vi "gyro calibration.vi"() -> ()   [LabVIEW 2012]
panel:
  in  "退出程序":bool caption="停止电机 2"
  out "角速度(deg/s)":dbl
  out "相对偏角(deg)":dbl(graph)
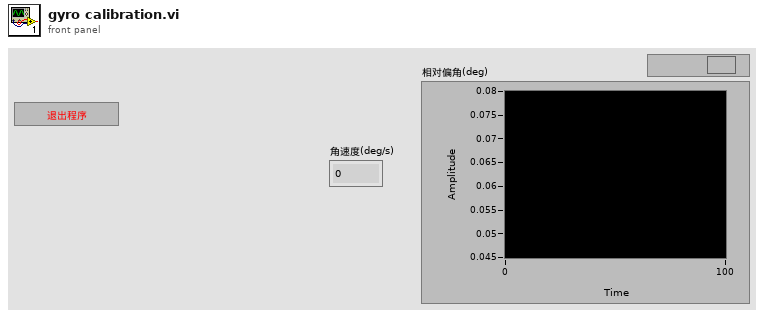
[diagram p1: front panel]
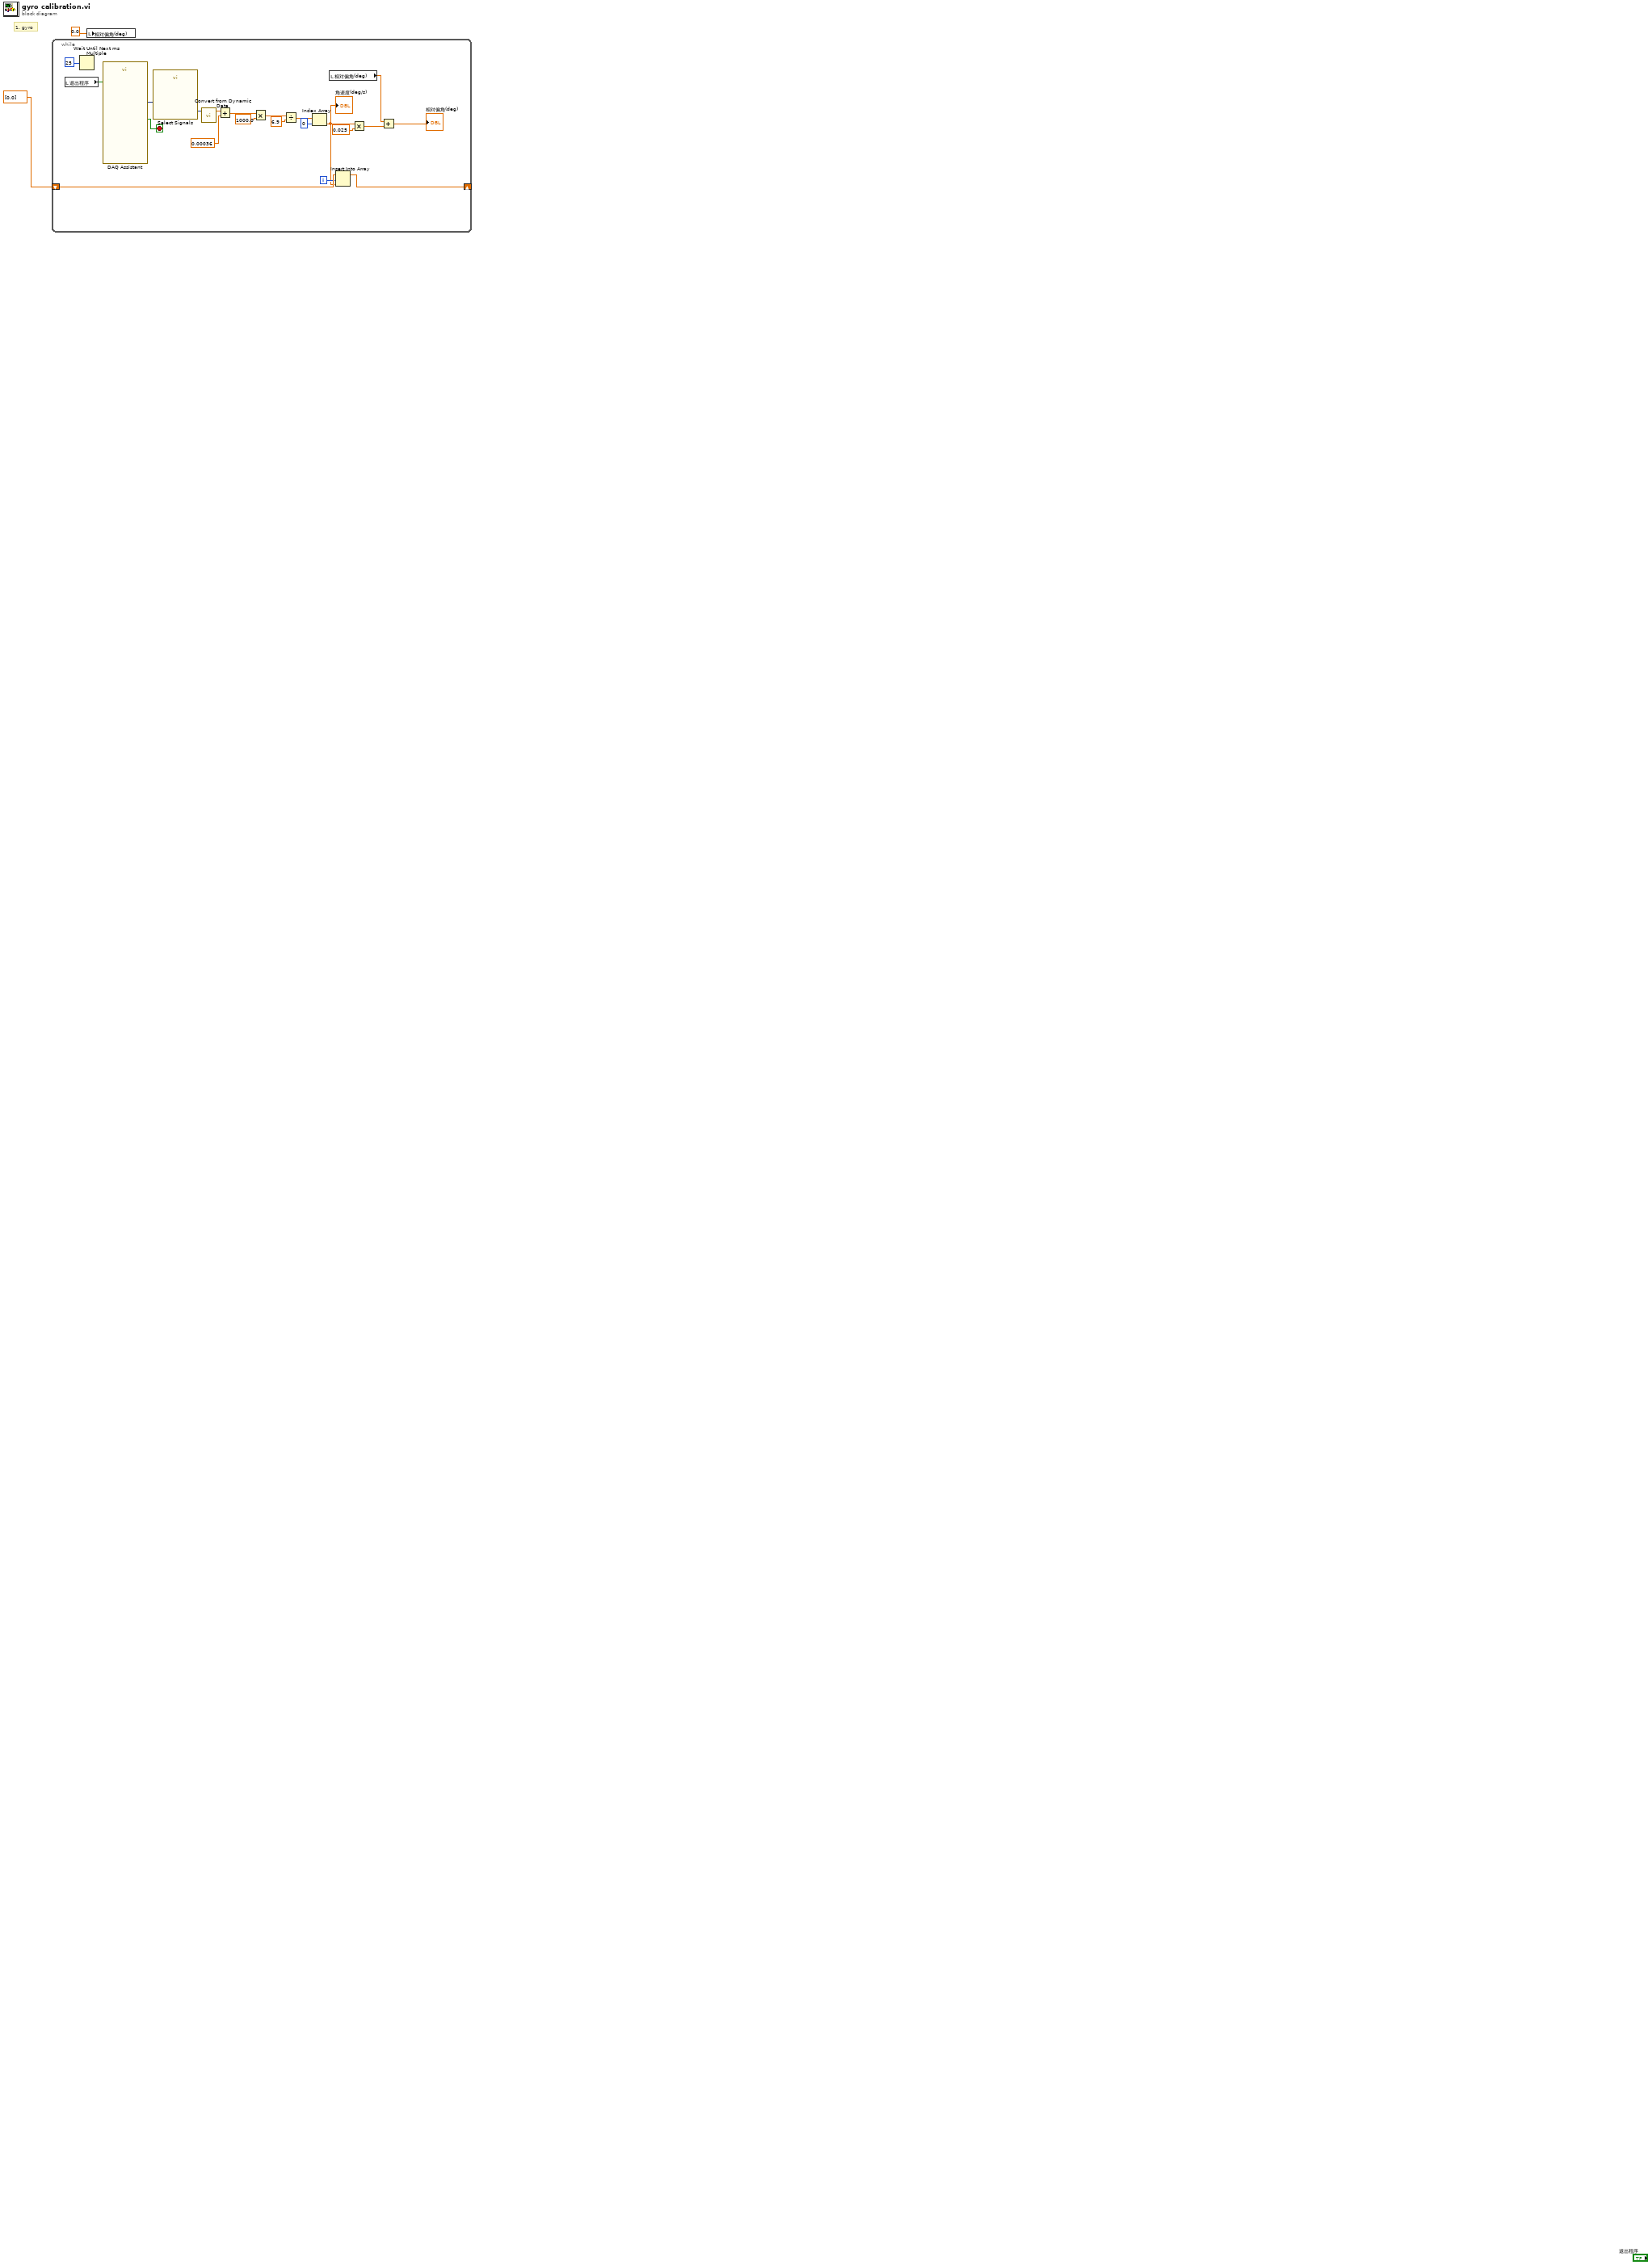
[diagram p0: block diagram]
diagram:
  # "1. gyro"
  n1 = while {
    shift-right: [w9] -> _
    shift-left: dbl[] [0.0] -> [w10]
    i -> [w8]
    stop <- w23 stop-if-true
    n2 = local read "退出程序"() -> (w6:bool)
    n3 = Wait Until Next ms Multiple(millisecond multiple=u32 25 ("y")) -> ()  [unwired: 1 out]
    n4 = call "DAQ Assistant"("stop (F)"=w6) -> ("data"=w4:dynamicdata, "stopped"=w23:bool)  [unwired: 15 in, 2 out]
    n5 = call "Select Signals"("Signals"=w4) -> ("Signal Out"=w5:dynamicdata)  [unwired: 9 in, 1 out]
    n6 = call "Convert from Dynamic Data"("Dynamic Data Type"=w5) -> ("Array"=w14:dbl[])  [unwired: 3 in]
    n7 = Add(x=w14, y=0.00036) -> (x+y=w12:dbl[])
    n8 = Multiply(x=w12, y=1000.0) -> (x*y=w22:dbl[])
    n9 = Divide(x=w22, y=6.9) -> (x/y=w16:dbl[])
    n10 = Index Array(array=w16, index=0) -> (element=w7:dbl)
    "角速度(deg/s)" <- w7
    n11 = local read "相对偏角(deg)"() -> (w11:dbl)
    n12 = Insert Into Array(array=w10, index=w8, new element=w7) -> (w9:dbl[])
    n13 = Multiply(x=w7, y=0.025) -> (x*y=w17:dbl)
    n14 = Add(x=w11, y=w17) -> (x+y=→"相对偏角(deg)":dbl)
  }
  n15 = local write "相对偏角(deg)"(0.0 ("y")) -> ()
